vi "fgt set custom Sensor Regulation.vi"(7 "pressureIndex":u32, 8 "error in (no error)":errorcluster, 9 "maxSensorRange":sgl, 10 "setpoint":sgl, 11 "measure":sgl) -> (0 "error out":errorcluster)   [LabVIEW 2017, in "fgt_SDK.lvlib"]
doc: "Start closed loop regulation between a sensor and a pressure controller. Pressure will be regulated in order to reach sensor setpoint.\nCustom sensors, outside Fluigent ones, can be used such as different flow-units, pressure, level ...\nHowever we do not guarantee full compatibility with all sensors. Regulation quality is linked to sensor precision and your set-up. Not supported by IPS.\nIn order to use this function, custom used sensor maximum range and measured values has to be updated at least once per second.\nDirectly setting pressure on same pressureIndex or not updating sensor value over 1s will stop regulation."
uses:
  fgt_SDK.lvlib
  dlls/fgt_SDK_32.dll
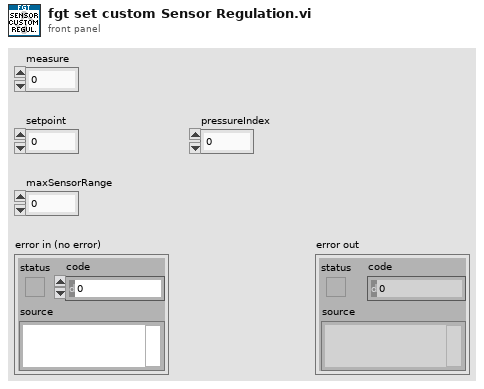
[diagram p1: front panel]
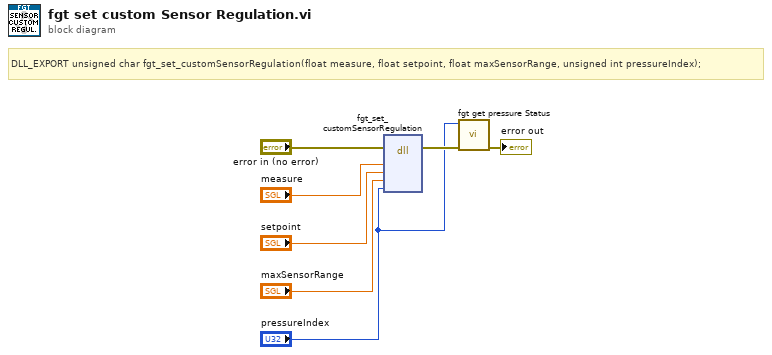
[diagram p0: block diagram]
diagram:
  # "DLL_EXPORT unsigned char fgt_set_customSensorRegulation(float measure, float setpoint, float maxSensorRange, unsigned int pressureIndex);"
  n1 = dll-call lib="D:/Work/SDK git/fgt-sdk-labview/dlls/fgt_SDK_*.*" fn="fgt_set_customSensorRegulation"(error in="error in (no error)", "measure"="measure", "setpoint"="setpoint", "maxSensorRange"="maxSensorRange", "pressureIndex"="pressureIndex") -> (error out=w3:errorcluster)  [unwired: 7 in, 1 out]
  n2 = call "fgt get pressure Status.vi"("error in (no error)"=w3, "pressureIndex"="pressureIndex") -> ("error out"=→"error out":errorcluster)  [unwired: 9 in]
